vi "Laser-response.vi"(8 "error in (no error)":errorcluster, 11 "Object ref in":T1) -> (0 "error out":errorcluster, 3 "Object ref out":T1)   [LabVIEW 2013, in "MaterialCharacterization.lvlib" / "MC-Main.lvclass"]
uses:
  MC-Main.lvclass
  Object-reference.ctl
  MC-Main.lvclass/MC-Main.ctl
  Read SM1000.vi
  Read Scan file path.vi
  Read LaserResponse.vi
  SM1000/MC-SM1000.lvclass
  LaserPulseAnalyser/MC-LaserResponse.lvclass
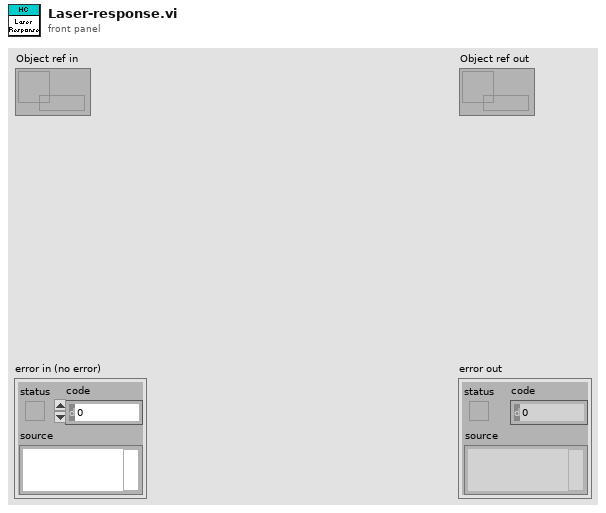
[diagram p1: front panel]
types:
  T1 = typedef "MaterialCharacterization.lvlib/MC-Main.lvclass/Object-reference.ctl" = refnum<data-value>
  T2 = typedef "MaterialCharacterization.lvlib/MC-SM1000.lvclass/Object-reference.ctl" = refnum<data-value>
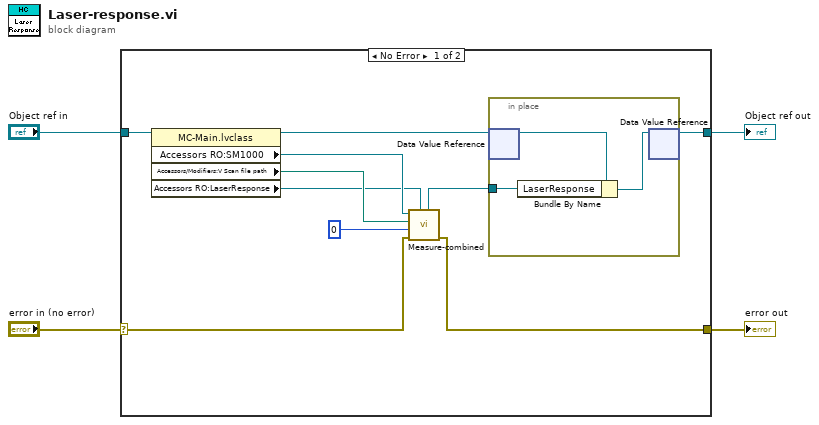
[diagram p0: block diagram]
diagram:
  n1 = case shown="No Error" "error in (no error)" {
    selector: "error in (no error)" -> [w10 w19]
    tunnel: [w9 w19] -> w3
    tunnel: [w7 w18] -> w1
    tunnel: "Object ref in" -> [w14 w18]
    frame No Error {
      n2 = property class="MC-Main.lvclass"(reference=w14) -> (reference out=w8:T1, "Accessors RO:SM1000"=w12:T2, "Accessors/Modifiers:V Scan file path"=w13:path, "Accessors RO:LaserResponse"=w6:refnum<class "MC-LaserResponse.lvclass">)  [unwired: 1 in, 1 out]
      n3 = call "Measure-combined.vi"("LaserResponse in"=w6, "error in (no error)"=w10, "Device index"=0, "File path"=w13, "SM1000-control in"=w12) -> ("error out"=w9:errorcluster, "LaserResponse"=w5:refnum<class "MC-LaserResponse.lvclass">)  [unwired: 4 in, 1 out]
      n4 = in-place {
        in-place-border: w5 -> [w15]
        n5 = in-place-dvr #1(w8) -> (w17:refnum<class "MC-Main.lvclass">)  [unwired: 1 out]
        n6 = Bundle By Name(cluster=w17, "LaserResponse"=w15) -> (w16:refnum<class "MC-Main.lvclass">)
        n7 = in-place-dvr #1(w16) -> (w7:T1)  [unwired: 1 out]
      }
    }
    frame Error {
    }
  }
  "error out" <- w3
  "Object ref out" <- w1
